vi "GetDSC.vi"(8 "error in (no error)":errorcluster, 11 "DSCNumber":u8) -> (0 "error out":errorcluster, 1 "LDSC board1":u32, 2 "ADSC board1":u32, 3 "LDSC board2":u32, 5 "ADSC board2":u32)   [LabVIEW 2015, in "ESLSCDLL.lvlib"]
uses:
  ESLSCDLL.lvlib
  Globals.vi
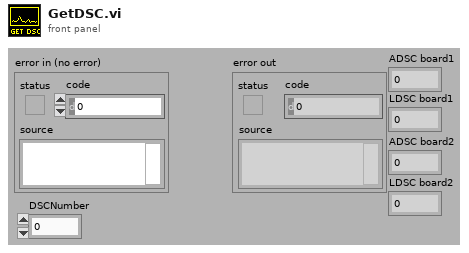
[diagram p1: front panel]
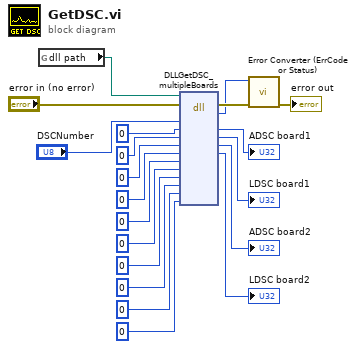
[diagram p0: block diagram]
diagram:
  n1 = global read "Globals.vi" "dll path"() -> (w1:path)
  n2 = dll-call lib="C:/ENTW/PCIE/LV64/board.vis/ESLSCDLL.dll" fn="DLLGetDSC_multipleBoards" ("lwlscdll.dll:DLLWriteLongS0")(path in=w1, error in="error in (no error)", "DSCNumber"="DSCNumber", "ADSC0"=u32 0 ("ADSC"), "LDSC0"=u32 0 ("LDSC"), "ADSC1"=u32 0, "LDSC1"=u32 0, "ADSC2"=u32 0, "LDSC2"=u32 0, "ADSC3"=u32 0, "LDSC3"=u32 0, "ADSC4"=u32 0, "LDSC4"=u32 0) -> (error out=w18:errorcluster, "es_status_codes"=w17:i32, "ADSC0"=→"ADSC board1":u32, "LDSC0"=→"LDSC board1":u32, "ADSC1"=→"ADSC board2":u32, "LDSC1"=→"LDSC board2":u32)  [unwired: 8 in, 1 out]
  n3 = call "Error Converter (ErrCode or Status).vi"("error in (no error)"=w18, "error code"=w17) -> ("error out"=→"error out":errorcluster)  [unwired: 9 in]
